vi "Update OD Category.vi"(8 "error in (no error)":errorcluster, 10 "file refnum":T1=refnum, 11 "Arr Refnum":refnum<vi>) -> (0 "error out":errorcluster, 3 "dup Arr Refnum":refnum<vi>)   [LabVIEW 2013]
uses:
  <vilib>/Utility/config.llb/Config Data RefNum.ctl
  control/OD Entry.ctl
  control/Object Type.ctl
  control/Data Type.ctl
  control/Access Type.ctl
  control/OD Cateory.ctl
  <vilib>/Utility/config.llb/NI_LVConfig.lvlib
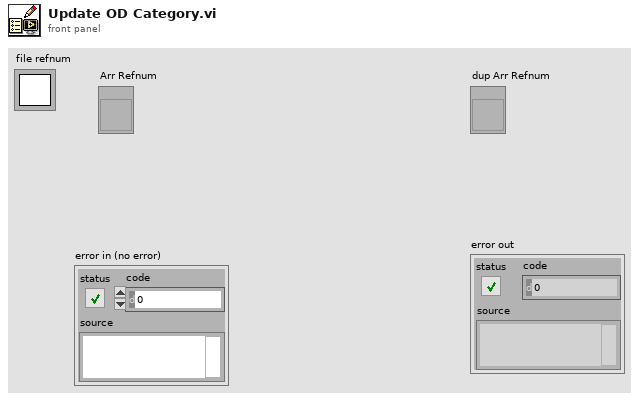
[diagram p1: front panel]
types:
  T1 = typedef "NI_LVConfig.lvlib/Config Data RefNum.ctl" = refnum<k1>
  T2 = typedef "OD Entry.ctl" = cluster{"index":u16, "sub-index":u8, "Level":u8, "ObjectType":T3, "DataType":T4, "ParameterName":string, "LowLimit":string, "HighLimit":string, "AccessType":T5, "DefaultValue":string, "PDOMapping":bool, "SubNumber":u8, "ObjFlags":u32, "Category":T6}
  T3 = typedef "Object Type.ctl" = u16
  T4 = typedef "Data Type.ctl" = u16
  T5 = typedef "Access Type.ctl" = u16
  T6 = typedef "OD Cateory.ctl" = enum16{"Mandatory", "Optional", "Manufacturer", ""}
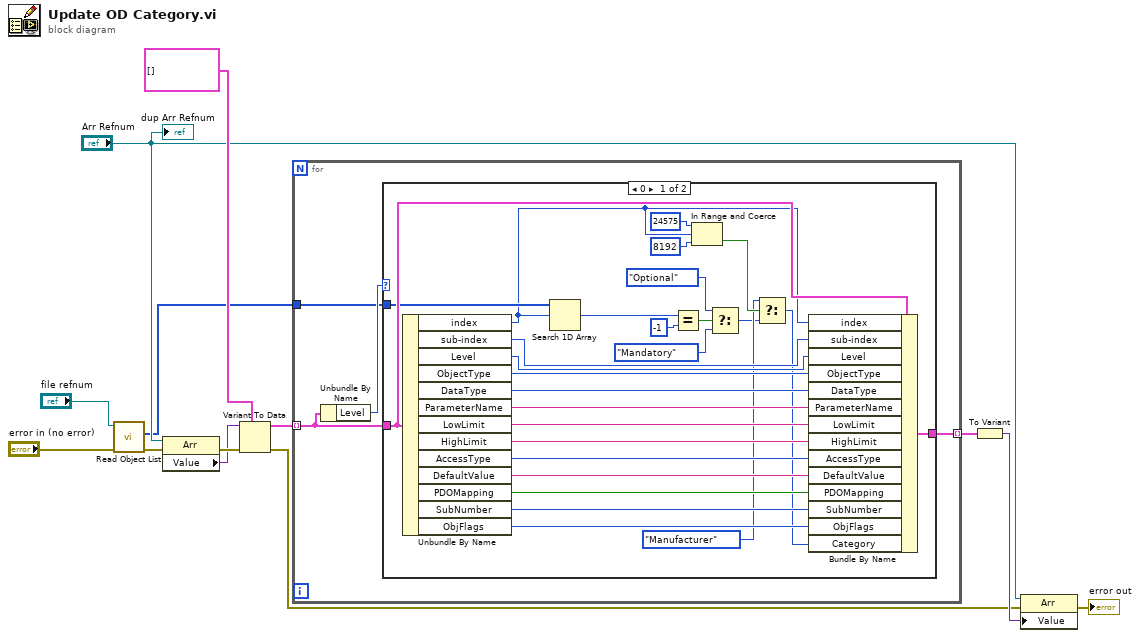
[diagram p0: block diagram]
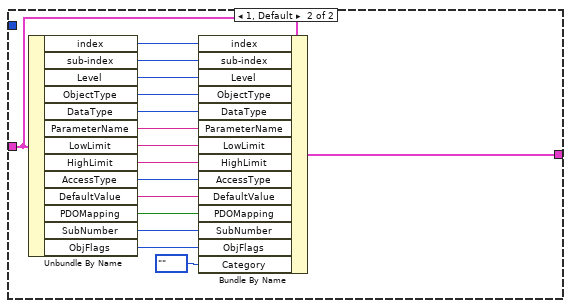
[diagram p2: hidden frame]
diagram:
  n1 = call "Read Object List.vi"("error in (no error)"="error in (no error)", "file refnum"="file refnum") -> ("error out"=w2:errorcluster, "Mandatory Object List"=w1:u16[])  [unwired: 7 in, 1 out]
  n2 = property class="Arr"(reference="Arr Refnum", error in=w2) -> (error out=w13:errorcluster, "Value"=w12:variant)  [unwired: 1 out]
  n3 = Variant To Data(error in=w13, type=T2[] [], Variant=w12) -> (data=w9:T2[], error out=w5:errorcluster)
  n4 = for {
    tunnel: w9 -> [w16] mode=indexing
    tunnel: [w15] -> w6 mode=indexing
    tunnel: w1 -> [w14]
    n5 = Unbundle By Name(w16) -> ("Level"=w17:u8)
    n6 = case shown="0" w17 {
      tunnel: w16 -> [w32 w47]
      tunnel: [w31 w45] -> w15
      tunnel: w14 -> [w25 _]
      frame 0 {
        n7 = Unbundle By Name(w32) -> ("index"=w24:u16, "sub-index"=w33:u8, "Level"=w34:u8, "ObjectType"=w35:T3, "DataType"=w36:T4, "ParameterName"=w37:string, "LowLimit"=w38:string, "HighLimit"=w39:string, "AccessType"=w40:T5, "DefaultValue"=w41:string, "PDOMapping"=w42:bool, "SubNumber"=w43:u8, "ObjFlags"=w44:u32)
        n8 = Search 1D Array(1D array=w25, element=w24) -> (index of element=w23:i32)  [unwired: 1 in]
        n9 = Equal?(x=w23, y=-1) -> (x = y?=w21:bool)
        n10 = In Range and Coerce(upper limit=u16 24575, x=w24, lower limit=u16 8192) -> (In Range?=w28:bool)  [unwired: 1 out]
        n11 = Select(t=OD_Cateory."Optional" ("f"), s=w21, f=OD_Cateory."Mandatory") -> (s? t:f=w19:T6)
        n12 = Select(t=OD_Cateory."Manufacturer" ("OD Cateory"), s=w28, f=w19) -> (s? t:f=w26:T6)
        n13 = Bundle By Name(cluster=w32, "index"=w24, "sub-index"=w33, "Level"=w34, "ObjectType"=w35, "DataType"=w36, "ParameterName"=w37, "LowLimit"=w38, "HighLimit"=w39, "AccessType"=w40, "DefaultValue"=w41, "PDOMapping"=w42, "SubNumber"=w43, "ObjFlags"=w44, "Category"=w26) -> (w31:T2)
      }
      frame 1, Default {
        n14 = Unbundle By Name(w47) -> ("index"=w48:u16, "sub-index"=w49:u8, "Level"=w50:u8, "ObjectType"=w51:T3, "DataType"=w52:T4, "ParameterName"=w53:string, "LowLimit"=w54:string, "HighLimit"=w55:string, "AccessType"=w56:T5, "DefaultValue"=w57:string, "PDOMapping"=w58:bool, "SubNumber"=w59:u8, "ObjFlags"=w60:u32)
        n15 = Bundle By Name(cluster=w47, "index"=w48, "sub-index"=w49, "Level"=w50, "ObjectType"=w51, "DataType"=w52, "ParameterName"=w53, "LowLimit"=w54, "HighLimit"=w55, "AccessType"=w56, "DefaultValue"=w57, "PDOMapping"=w58, "SubNumber"=w59, "ObjFlags"=w60, "Category"=OD_Cateory."") -> (w45:T2)
      }
    }
  }
  n16 = To Variant(anything=w6) -> (Variant=w7:variant)
  n17 = property class="Arr"(reference="Arr Refnum", error in=w5, "Value"=w7) -> (error out=→"error out":errorcluster)  [unwired: 1 out]
  "dup Arr Refnum" <- "Arr Refnum"
